vi "PID_2_Channels.vi"() -> ()   [LabVIEW 2016]
uses:
  <vilib>/addons/control/pid/pid.llb/PID Advanced (DBL Array).vi
  <vilib>/Analysis/baseanly.llb/Mean (DBL).vi
  <vilib>/addons/control/pid/pid.llb/PID Parameter Manager (DBL Array).vi
  <vilib>/addons/control/pid/pid.llb/PID Derivative Action Buffered (DBL Array).vi
  <vilib>/addons/control/pid/pid.llb/PID Get Advanced Error (DBL Array).vi
  <vilib>/addons/control/pid/pid.llb/PID Integral Action Buffered (DBL Array).vi
  <vilib>/addons/control/pid/pid.llb/PID Resize 1D Array.vi
  <vilib>/addons/control/pid/pid.llb/PID Get Advanced Error (DBL).vi
  <userlib>/Fluigent/Fluigent MFCS/FluigentMFCS_Full.llb/MFCS_EZ Detect.vi
  <userlib>/Fluigent/Fluigent MFCS/FluigentMFCS_Full.llb/MFCS_EZ Initialization.vi
  <userlib>/Fluigent/Fluigent MFCS/FluigentMFCS_Full.llb/MFCS_EZ Read Channel Pressure.vi
  <userlib>/Fluigent/Fluigent MFCS/FluigentMFCS_Full.llb/MFCS_EZ Write Channel Pressure.vi
  <vilib>/addons/control/pid/NI_PID_autopid.lvlib
  <vilib>/Analysis/NI_AALBase.lvlib
  <vilib>/addons/control/pid/NI_PID_pid.lvlib
  <vilib>/addons/control/pid/autopid.llb/PID Autotuning Design (Auto).vi
panel:
  out "F0":dbl[](graph)
  out "Flow Setpoints":dbl[](array[numeric])
  in  "Manual Total Mix Flow":dbl
  out "Total Mix Flow":dbl
  in  "Ratio":dbl
  in  "Add Ctrl?":bool
  in  "output range":cluster{"output high":dbl, "output low":dbl}[](array[cluster])=[{"output high"=1200.0, "output low"=0.0}] {"output low" format="%.2f"; "output high" format="%.2f"}
  out "x-y":dbl=-11785.0
  out "X Scale.Range:Minimum":dbl=253481745.0
  out "X Scale.Range:Maximum":dbl=253469960.0
  out "Flow Rate 2":dbl[](graph)
  in  "setpoint range":T1(array[cluster])=[{"setpoint high"=100.0, "setpoint low"=0.0}] {"setpoint high" format="%.2f"; "setpoint low" format="%.2f"}
  out "Tuning Completed":bool[](array[boolean])
  out "Tuned Gains":T2(array[cluster])
  in  "Manual Pressure Set":dbl[](array[numeric])=[300.0, 310.0]
  in  "Pressure Channels":enum16{"1", "2", "3", "4"}[](array[ring])=[enum."1", enum."2"]
  out "Feedback Sig":dbl[][](graph)
  in  "gamma":dbl[](array[numeric])=[0.0] format="%.2f"
  in  "linearity":dbl[](array[numeric])=[1.0] format="%.2f"
  in  "beta":dbl[](array[numeric])=[1.0] format="%.2f"
  in  "PID Gains":T3(array[cluster])=[{"Proportional Gain"=0.5, "Integral Time"=0.01, "Derivative Time"=0.0}, {"Proportional Gain"=0.5, "Integral Time"=0.01, "Derivative Time"=0.0}]
  in  "Fwater":dbl
  out "Current F2":dbl=98.13793103448276
  out "Current F0":dbl=248.41379310344828
  in  "Valves":enum16{"1", "2", "3", "4", "5", "6", "7", "8"}[](array[ring])=[enum."5", enum."1"]
  in  "Boards":enum16{"A", "B", "C"}[](array[ring])=[enum."A", enum."A"]
  out "error out":errorcluster
  out "dt":dbl=0.024001121520996094
  in  "Filter Size":i32=5
  out "Filtered Flow":dbl=150.2206896551724 format="%0.2f"
  out "Current F1":dbl=150.27586206896552
  in  "reinitialize? (F)":bool
  out "response operating point":dbl
  out "stimulus operating point":dbl
  in  "Control on":bool=TRUE
  out "Flow Rate 1":dbl[](graph)
  out "Pressure Setpoint":dbl[][](graph)
  in  "stop":bool
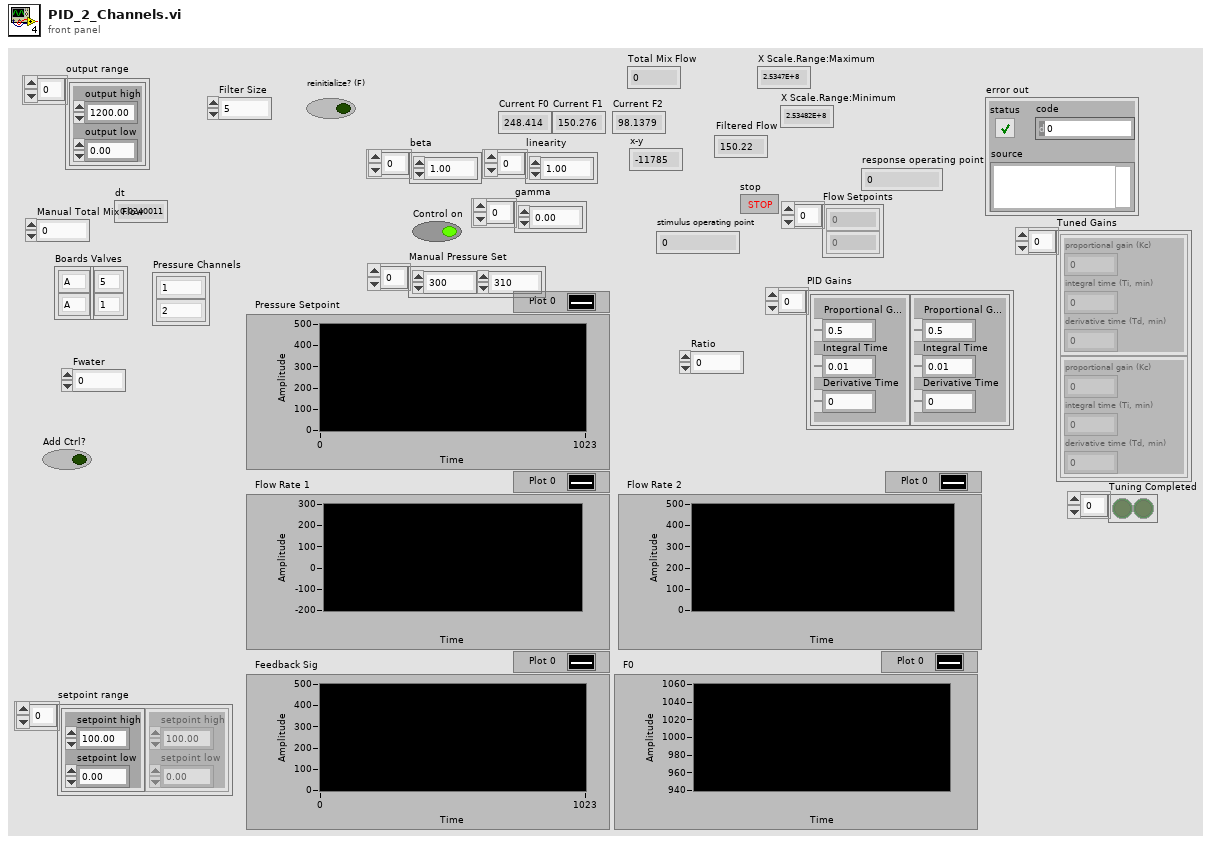
[diagram p1: front panel]
types:
  T1 = cluster{"setpoint high":dbl, "setpoint low":dbl}[]
  T2 = cluster{"proportional gain (Kc)":dbl, "integral time (Ti, min)":dbl, "derivative time (Td, min)":dbl}[]
  T3 = cluster{"Proportional Gain":dbl, "Integral Time":dbl, "Derivative Time":dbl}[]
  T4 = typedef "_EZmfcsSN.ctl" = u16
  T5 = typedef "_frpRefNum" = refnum<k1>
  T6 = typedef "_EZmfcsRefNum.ctl" = refnum<k1>
  T7 = cluster{"proportional gain (Kc)":dbl, "integral time (Ti, min)":dbl, "derivative time (Td, min)":dbl}
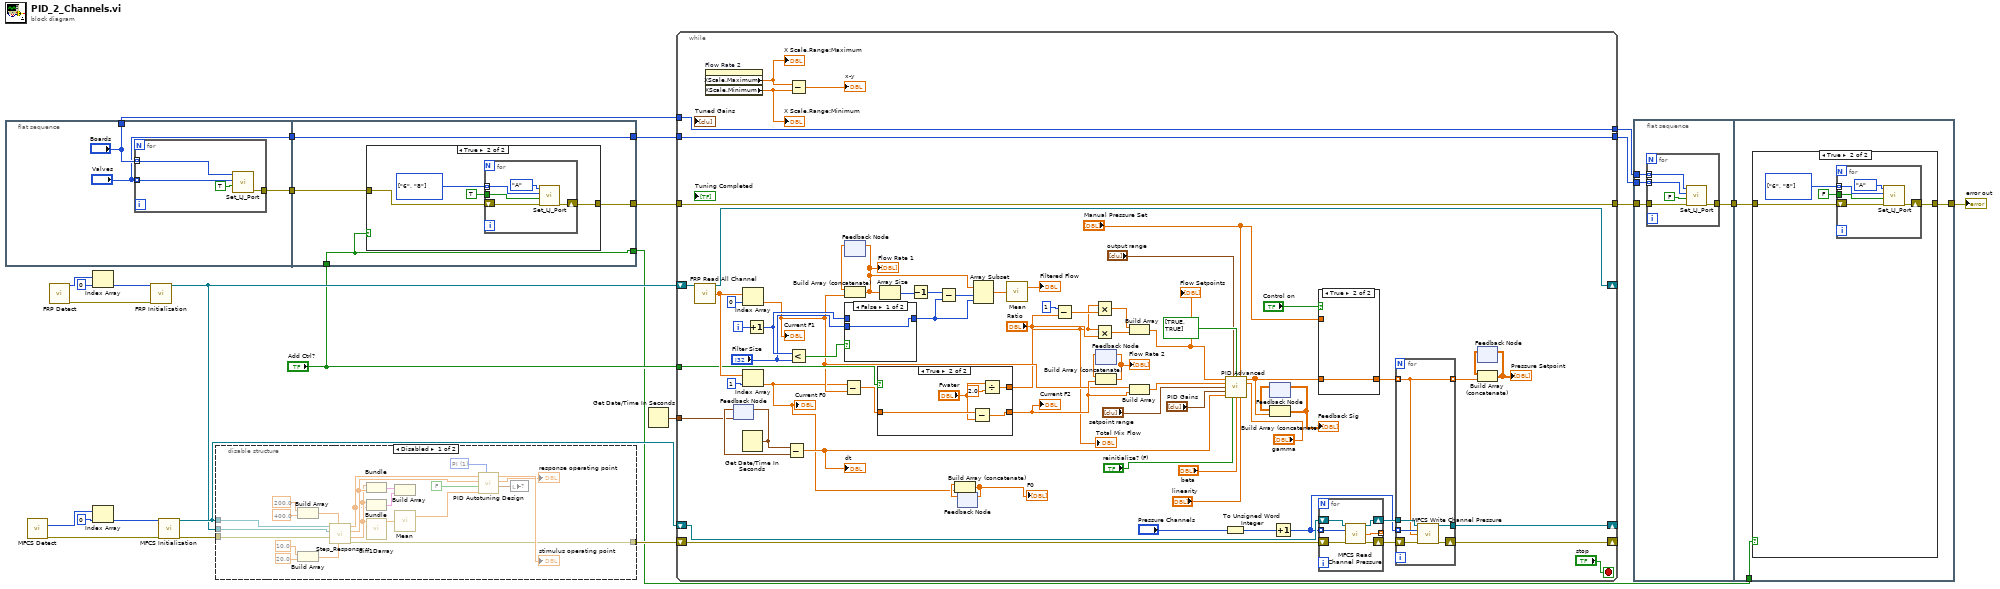
[diagram p0: block diagram]
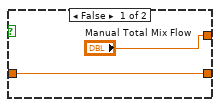
[diagram p5: hidden frame]
diagram:
  n1 = flat-sequence {
    tunnel: ["Boards"] -> w11
    tunnel: [w28] -> w5
    tunnel: ["Valves"] -> w4
    tunnel: [w36] -> w10
    tunnel: [w34] -> w12
    tunnel: w5 -> [w35]
    tunnel: w4 -> [w36]
    tunnel: "Add Ctrl?" -> [w33]
    tunnel: [w33] -> w1
    frame #0 {
      n2 = for {
        tunnel: "Valves" -> [w32] mode=indexing
        tunnel: "Boards" -> [w31] mode=indexing
        tunnel: [w29] -> w28
        n3 = call "Set_LJ_Port.vi"("State"=TRUE, "Channel"=w32, "Flowboard"=w31) -> ("error out"=w29:errorcluster)  [unwired: 8 in]
      }
    }
    frame #1 {
      n4 = case shown="True" w33 {
        tunnel: w35 -> [w37 w41]
        tunnel: [w37 w40] -> w34
        frame False {
        }
        frame True {
          w38 = enum16{"1", "2", "3", "4", "5", "6", "7", "8"}[] [enum."6", enum."8"] items=["1", "2", "3", "4", "5", "6", "7", "8"]
          n5 = for {
            tunnel: TRUE ("State") -> [w44]
            shift-right: [w45] -> w40
            shift-left: w41 -> [w46]
            tunnel: w38 -> [w43] mode=indexing
            n6 = call "Set_LJ_Port.vi"("error in"=w46, "State"=w44, "Channel"=w43, "Flowboard"=enum16{"A", "B", "C"}."A") -> ("error out"=w45:errorcluster)  [unwired: 7 in]
          }
        }
      }
    }
  }
  n7 = call-poly <userlib>:"MFCS Detect.vi"() -> ("[SN MFCS_EZ]"=w25:T4[], "error out"=w23:errorcluster)  [unwired: 14 in]
  n8 = call <userlib>:"FRP Detect.vi"() -> ("FLOWBOARD List"=w22:u16[], "error out"=w19:errorcluster)  [unwired: 14 in]
  n9 = Index Array(array=w22, index=0) -> (element=w18:u16)
  n10 = Index Array(array=w25, index=0) -> (element=w24:T4)
  n11 = call <userlib>:"FRP Initialization.vi"("Serial Number"=w18, "error in (no error)"=w19) -> ("FRP out"=w16:T5)  [unwired: 11 in, 2 out]
  n12 = call-poly <userlib>:"MFCS Initialization.vi"("SN MFCS_EZ"=w24, "error in (no error)"=w23) -> ("MFCS_EZ"=w17:T6, "error out"=w14:errorcluster)  [unwired: 11 in, 1 out]
  n13 = disable-structure shown="Disabled" {
    disable-tunnel: w17 -> [w68 _]
    disable-tunnel: w16 -> [w67 _]
    disable-tunnel: [w59 w69] -> w15
    disable-tunnel: w14 -> [w58 w69]
    frame Disabled {
      w63 = u16 1 items=["P", "PI", "PID"] ("Type of Controller")
      n14 = Build Array(200.0 ("element"), 400.0 ("element")) -> (w51:dbl[])
      n15 = Build Array(10.0 ("element"), 20.0 ("element")) -> (w52:dbl[])
      n16 = call "Step_Response.vi"("Times"=w52, "Pressure Sets"=w51, "MFCS Error"=w58, "FRP Handle"=w67, "MFCS Handle"=w68) -> ("error out"=w59:errorcluster, "T"=w50:dbl[], "Flow Rate"=w53:dbl[], "Pressure Setpoint"=w49:dbl[])  [unwired: 3 in]
      n17 = Bundle("T"=w50, "Flow Rate"=w53) -> (w47:cluster{"T":dbl[], "Flow Rate":dbl[]})  [unwired: 1 in]
      n18 = Bundle("T"=w50, "Pressure Setpoint"=w49) -> (w48:cluster{"T":dbl[], "Pressure Setpoint":dbl[]})  [unwired: 1 in]
      n19 = call "diff1Darray.vi"("Input"=w50) -> ("Diff"=w65:dbl[])  [unwired: 10 in]
      n20 = Build Array(w47, w48) -> ()  [unwired: 1 out]
      n21 = call-poly <vilib>:"Mean.vi"("X"=w65) -> ("mean"=w64:dbl)  [unwired: 1 out]
      n22 = call-poly <vilib>:"PID Autotuning Design.vi"("Type of Controller"=w63, "dt (s)"=w64, "closed-loop?"=FALSE, "Response signal"=w53, "Stimulus signal"=w49) -> ("PID gains"=w62:T7, "response operating point"=→"response operating point":dbl, "stimulus operating point"=→"stimulus operating point":dbl)  [unwired: 3 in, 1 out]
      n23 = local write item#-1(w62) -> ()
    }
    frame Enabled {
    }
  }
  n24 = Get Date/Time In Seconds() -> (seconds since 1Jan1904=w13:timestamp)
  n25 = while {
    shift-right: [w113] -> _
    shift-left: w15 -> [w139]
    shift-right: [w110] -> _
    shift-left: w17 -> [w140]
    shift-right: [w136] -> _
    shift-left: w16 -> [w137]
    tunnel: [w118] -> w7
    tunnel: w12 -> [w118]
    tunnel: w13 -> [w101]
    tunnel: w11 -> [w119]
    tunnel: w10 -> [w120]
    tunnel: [w120] -> w9
    tunnel: [w119] -> w8
    tunnel: "Add Ctrl?" -> [w81]
    i -> [w131]
    stop <- "stop" stop-if-true
    n26 = call <userlib>:"FRP Read All Channel.vi"("FRP"=w137) -> ("FRP out"=w136:T5, "All Flow-Rates"=w116:dbl[])  [unwired: 12 in, 1 out]
    n27 = property on="Flow Rate 2" class="WFChart (strict)"() -> ("XScale.Maximum"=w98:dbl, "XScale.Minimum"=w97:dbl)  [unwired: 2 in, 2 out]
    "X Scale.Range:Maximum" <- w98
    "X Scale.Range:Minimum" <- w97
    n28 = feedback #1(w101) -> (w132:timestamp)
    n29 = Get Date/Time In Seconds() -> (seconds since 1Jan1904=w133:timestamp)
    n30 = feedback-in #1(w133) -> ()
    n31 = Index Array(array=w116, index=0) -> (element=w80:dbl)
    "Current F1" <- w80
    n32 = Index Array(array=w116, index=1) -> (element=w70:dbl)
    "Current F0" <- w70
    n33 = Increment(x=w131) -> (x+1=w129:i32)
    n34 = Subtract(x=w133, y=w132) -> (x-y=w107:dbl)
    "dt" <- w107
    n35 = Subtract(x=w98, y=w97) -> (x-y=→"x-y":dbl)
    n36 = Less?(x=w129, y="Filter Size") -> (x < y?=w130:bool)
    n37 = Subtract(x=w70, y=w80) -> (x-y=w83:dbl)
    n38 = feedback #2() -> (w134:dbl[])  [unwired: 1 in]
    n39 = Build Array (concatenate)(w134, w80) -> (w124:dbl[])
    "Flow Rate 1" <- w124
    n40 = feedback-in #2(w124) -> ()
    n41 = case shown="False" w130 {
      tunnel: w129 -> [_ w163]
      tunnel: [w162 w163] -> w126
      tunnel: "Filter Size" -> [w162 _]
      frame False {
      }
      frame True {
      }
    }
    n42 = case shown="True" w81 {
      tunnel: w83 -> [w142 w147]
      tunnel: [w142 w146] -> w82
      tunnel: ["Manual Total Mix Flow" w143] -> w75
      frame False {
      }
      frame True {
        n43 = Subtract(x=w147, y="Fwater") -> (x-y=w146:dbl)
        n44 = Divide(x="Fwater", y=2.0) -> (x/y=w143:dbl)
      }
    }
    "Current F2" <- w82
    "Total Mix Flow" <- w75
    n45 = Array Size(array=w124) -> (size(s)=w127:i32)
    n46 = Decrement(x=w127) -> (x-1=w125:i32)
    n47 = Subtract(x=w125, y=w126) -> (x-y=w123:i32)
    n48 = feedback #3() -> (w71:dbl[])  [unwired: 1 in]
    n49 = Build Array (concatenate)(w71, w70) -> (w72:dbl[])
    "F0" <- w72
    n50 = feedback-in #3(w72) -> ()
    n51 = Array Subset(array=w124, index=w123, length=w126) -> (w122:dbl[])
    n52 = call-poly <vilib>:"Mean.vi"("X"=w122) -> ("mean"=→"Filtered Flow":dbl)  [unwired: 1 out]
    n53 = Subtract(x=1, y="Ratio") -> (x-y=w78:dbl)
    n54 = Multiply(x=w75, y=w78) -> (x*y=w77:dbl)
    n55 = Multiply(x=w75, y="Ratio") -> (x*y=w74:dbl)
    n56 = feedback #4() -> (w100:dbl[])  [unwired: 1 in]
    n57 = Build Array (concatenate)(w100, w82) -> (w99:dbl[])
    "Flow Rate 2" <- w99
    n58 = feedback-in #4(w99) -> ()
    n59 = Build Array(w77, w74) -> (w73:dbl[])
    "Flow Setpoints" <- w73
    n60 = Build Array(w80, w82) -> (w85:dbl[])
    n61 = To Unsigned Word Integer(number="Pressure Channels") -> (unsigned 16bit integer=w95:u16[])
    n62 = call-poly <vilib>:"PID Advanced.vi"("setpoint"=w73, "output range"="output range", "auto? (T)"=bool[] [TRUE, TRUE] ("appended array"), "manual control"="Manual Pressure Set", "process variable"=w85, "gamma"="gamma", "setpoint range"="setpoint range", "PID gains"="PID Gains", "dt (s)"=w107, "reinitialize? (F)"="reinitialize? (F)", "beta"="beta", "linearity"="linearity") -> ("output"=w88:dbl[])  [unwired: 2 in, 1 out]
    n63 = feedback #5() -> (w94:dbl[][])  [unwired: 1 in]
    n64 = Build Array (concatenate)(w94, w88) -> (w93:dbl[][])
    "Feedback Sig" <- w93
    n65 = feedback-in #5(w93) -> ()
    n66 = Increment(x=w95) -> (x+1=w102:u16[])
    n67 = case shown="True" "Control on" {
      tunnel: "Manual Pressure Set" -> [w148 _]
      tunnel: [w148 w149] -> w89
      tunnel: w88 -> [_ w149]
      frame False {
      }
      frame True {
      }
    }
    n68 = for {
      tunnel: [w153] -> _ mode=indexing
      shift-right: [w152] -> w115
      shift-left: w140 -> [w155]
      shift-right: [w151] -> w114
      shift-left: w139 -> [w154]
      tunnel: w102 -> [w150] mode=indexing
      n69 = call-poly <userlib>:"MFCS Read Channel Pressure.vi"("MFCS_EZ"=w155, "Channel Number (default=1)"=w150, "error in (no error)"=w154) -> ("MFCS_EZ out"=w152:T6, "Pressure (mBar)"=w153:dbl, "error out"=w151:errorcluster)  [unwired: 9 in, 1 out]
    }
    n70 = for {
      tunnel: w115 -> [w161]
      shift-right: [w159] -> w113
      shift-left: w114 -> [w160]
      tunnel: [w156] -> w86 mode=indexing
      tunnel: [w158] -> w110
      tunnel: w102 -> [w157] mode=indexing
      tunnel: w89 -> [w156] mode=indexing
      n71 = call-poly <userlib>:"MFCS Write Channel Pressure.vi"("MFCS_EZ"=w161, "Channel Number (default=1)"=w157, "Pressure (mBar)"=w156, "error in (no error)"=w160) -> ("MFCS_EZ out"=w158:T6, "error out"=w159:errorcluster)  [unwired: 10 in]
    }
    n72 = feedback #6() -> (w112:dbl[][])  [unwired: 1 in]
    n73 = Build Array (concatenate)(w112, w86) -> (w111:dbl[][])
    "Pressure Setpoint" <- w111
    n74 = feedback-in #6(w111) -> ()
  }
  n75 = flat-sequence {
    tunnel: w9 -> [w167]
    tunnel: w8 -> [w166]
    tunnel: w7 -> [w165]
    tunnel: [w164] -> w2
    tunnel: [w174] -> w6
    tunnel: w2 -> [w173]
    tunnel: w1 -> [w175]
    frame #0 {
      n76 = for {
        tunnel: w167 -> [w172] mode=indexing
        tunnel: [w170] -> w164
        tunnel: w166 -> [w169] mode=indexing
        tunnel: w165 -> [w168]
        n77 = call "Set_LJ_Port.vi"("error in"=w168, "State"=FALSE, "Channel"=w172, "Flowboard"=w169) -> ("error out"=w170:errorcluster)  [unwired: 7 in]
      }
    }
    frame #1 {
      n78 = case shown="True" w175 {
        tunnel: w173 -> [w176 w177]
        tunnel: [w176 w180] -> w174
        frame False {
        }
        frame True {
          w178 = enum16{"1", "2", "3", "4", "5", "6", "7", "8"}[] [enum."6", enum."8"] items=["1", "2", "3", "4", "5", "6", "7", "8"]
          n79 = for {
            tunnel: FALSE ("State") -> [w183]
            shift-right: [w184] -> w180
            shift-left: w177 -> [w185]
            tunnel: w178 -> [w182] mode=indexing
            n80 = call "Set_LJ_Port.vi"("error in"=w185, "State"=w183, "Channel"=w182, "Flowboard"=enum16{"A", "B", "C"}."A") -> ("error out"=w184:errorcluster)  [unwired: 7 in]
          }
        }
      }
    }
  }
  "error out" <- w6
